vi "demo_idn.vi"() -> ()   [LabVIEW 2017]
panel:
  out "IDN":string
  in  "name":string="mrx-t4"
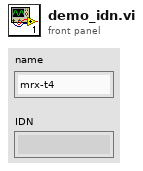
[diagram p1: front panel]
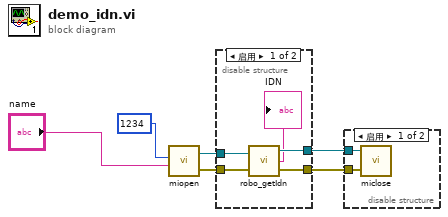
[diagram p0: block diagram]
diagram:
  n1 = call "miopen.vi"("name"="name", "port"=u16 1234) -> ("错误输出"=w3:errorcluster, "VISA资源名称输出"=w6:refnum<visa-resource-name>)  [unwired: 2 in]
  n2 = disable-structure shown="启用" {
    disable-tunnel: w6 -> [w11 w13]
    disable-tunnel: [w10 w13] -> w5
    disable-tunnel: [w9 w12] -> w4
    disable-tunnel: w3 -> [w8 w12]
    frame Enabled {
      n3 = call "robo_getIdn.vi"("VISA资源名称"=w11, "错误输入（无错误）"=w8) -> ("VISA资源名称输出"=w10:refnum<visa-resource-name>, "读取缓冲区"=→"IDN":string, "错误输出"=w9:errorcluster)
    }
    frame Disabled {
    }
  }
  n4 = disable-structure shown="启用" {
    disable-tunnel: w5 -> [w15 _]
    disable-tunnel: w4 -> [w14 _]
    frame Enabled {
      n5 = call "miclose.vi"("错误输入（无错误）"=w14, "VISA资源名称"=w15) -> ()  [unwired: 1 out]
    }
    frame Disabled {
    }
  }
